vi "acquisitionSaveBuffer.vi"   [LabVIEW 2017]
uses:
  globalDevices.vi
  globalUtilities.vi
types:
  T1 = enum16{"big-endian, network order", "native, host order", "little-endian"}
  T2 = enum16{"open", "replace", "create", "open or create", "replace or create", "replace or create with confirmation"}
  T3 = cluster{"height":i32, "width":i32, "datatype":i32}
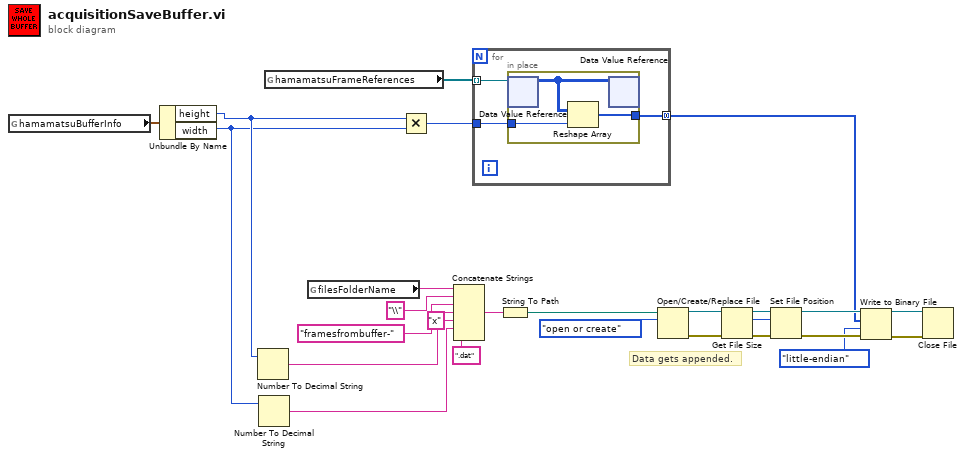
[diagram p0: block diagram]
diagram:
  # "Data gets appended."
  n1 = global read "globalDevices.vi" "hamamatsuBufferInfo"() -> (w25:T3)
  n2 = Unbundle By Name(w25) -> ("height"=w20:i32, "width"=w19:i32)
  n3 = Number To Decimal String(number=w20) -> (decimal integer string=w18:string)  [unwired: 1 in]
  n4 = Number To Decimal String(number=w19) -> (decimal integer string=w16:string)  [unwired: 1 in]
  n5 = global read "globalDevices.vi" "hamamatsuFrameReferences"() -> (w26:refnum<data-value>[])
  n6 = global read "globalUtilities.vi" "filesFolderName"() -> (w23:string)
  n7 = Multiply(x=w20, y=w19) -> (x*y=w24:i32)
  n8 = Concatenate Strings(w23, "\\" ("string"), "framesfrombuffer-" ("string"), w18, "x" ("string"), w16, ".dat" ("string")) -> (w14:string)
  n9 = for {
    tunnel: w26 -> [w29] mode=indexing
    tunnel: w24 -> [w28]
    tunnel: [w27] -> w3 mode=concatenating
    n10 = in-place {
      in-place-border: w28 -> [w31]
      in-place-border: [w30] -> w27
      n11 = in-place-dvr #1(w29) -> (w32:u16[][])  [unwired: 1 out]
      n12 = Reshape Array(w32, w31) -> (w30:u16[])
      n13 = in-place-dvr #1(w32) -> ()  [unwired: 2 out]
    }
  }
  n14 = String To Path(string=w14) -> (path=w13:path)
  n15 = Open/Create/Replace File(file path (use dialog)=w13, operation (0:open)=T2."open or create") -> (refnum out=w11:refnum<file>, error out=w10:errorcluster)  [unwired: 4 in, 1 out]
  n16 = Get File Size(file=w11, error in=w10) -> (refnum out=w9:refnum<file>, size (in bytes)=w7:i64, 0:w8:errorcluster)
  n17 = Set File Position(offset (in bytes) (0)=w7, refnum=w9, error in=w8) -> (refnum out=w6:refnum<file>, error out=w5:errorcluster)  [unwired: 1 in]
  n18 = Write to Binary File(file (use dialog)=w6, data=w3, error in=w5, 9:T1."little-endian" ("byte order (0:big-endian, network order)")) -> (refnum out=w2:refnum<file>, error out=w1:errorcluster)  [unwired: 2 in, 1 out]
  n19 = Close File(refnum=w2, error in=w1) -> ()  [unwired: 2 out]
